vi "RT Init FAST Arrays.vi"() -> (1 "FAST array":sgl[](array[numeric]), 2 "Blade Array":sgl[](array[numeric]))   [LabVIEW 2012]
panel:
  # "This VI creates FIFOs and array\nfor use in FAST simulation"
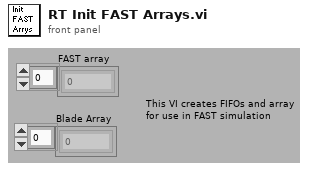
[diagram p1: front panel]
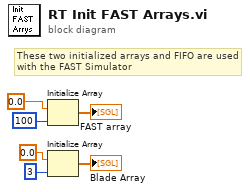
[diagram p0: block diagram]
diagram:
  # "These two initialized arrays and FIFO are used\nwith the FAST Simulator"
  n1 = Initialize Array(sgl 0.0 ("element"), 100 ("dimension size")) -> (→"FAST array":sgl[])
  n2 = Initialize Array(sgl 0.0 ("element"), 3 ("dimension size")) -> (→"Blade Array":sgl[])
